vi "Transfer Properties to New Node.vi"(7 "Replacement Channels":T1={"Channel to Replace"="Targets/Controller/Custom Devices/VCOM/CAN_Sender_Tx/ACC/ACC_ESP_E2E_PR2/ACC_NEW_SIGNAL", "Replacement Channel"="Targets/Controller/User Channels/User Channel 1"}, 8 "error in (no error)":errorcluster, 10 "Property Type":i32(ring)=8 items=["K_STRING", "K_BOOL", "K_I32", "K_U32", "K_DOUBLE", "K_U64", "K_VARIANT", "K_DEPENDENTFILE", "K_DEPENDENTNODE", "K_DATASOURCENODE", "K_U16", "K_DBLARR", "K_U32ARR", "K_I32ARR", "K_STRINGARR", "K_DICTIONARY", "K_DICTIONARYARR", "K_BINARYSTRING", "K_I16", "K_I64", "K_BOOLARR", "K_U64ARR", "K_U16ARR", "K_I64ARR", "K_I16ARR"], 11 "reference":refnum<k24>) -> (0 "error out":errorcluster, 2 "Replacement Log":string[](array[string]), 3 "reference out":refnum<k24>)   [LabVIEW 2025]
uses:
  Replacement Channels.ctl
  NationalInstruments.VeriStand.SystemDefinitionAPI
  NationalInstruments.VeriStand.SystemStorage
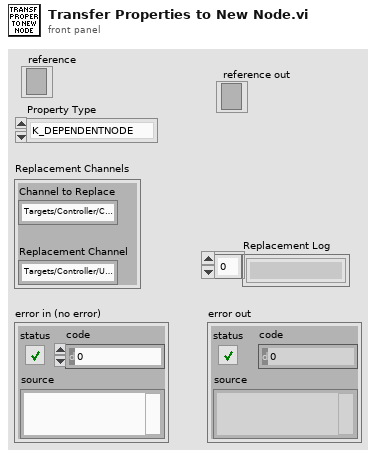
[diagram p1: front panel]
types:
  T1 = typedef "Replacement Channels.ctl" = cluster{"Channel to Replace":string, "Replacement Channel":string}
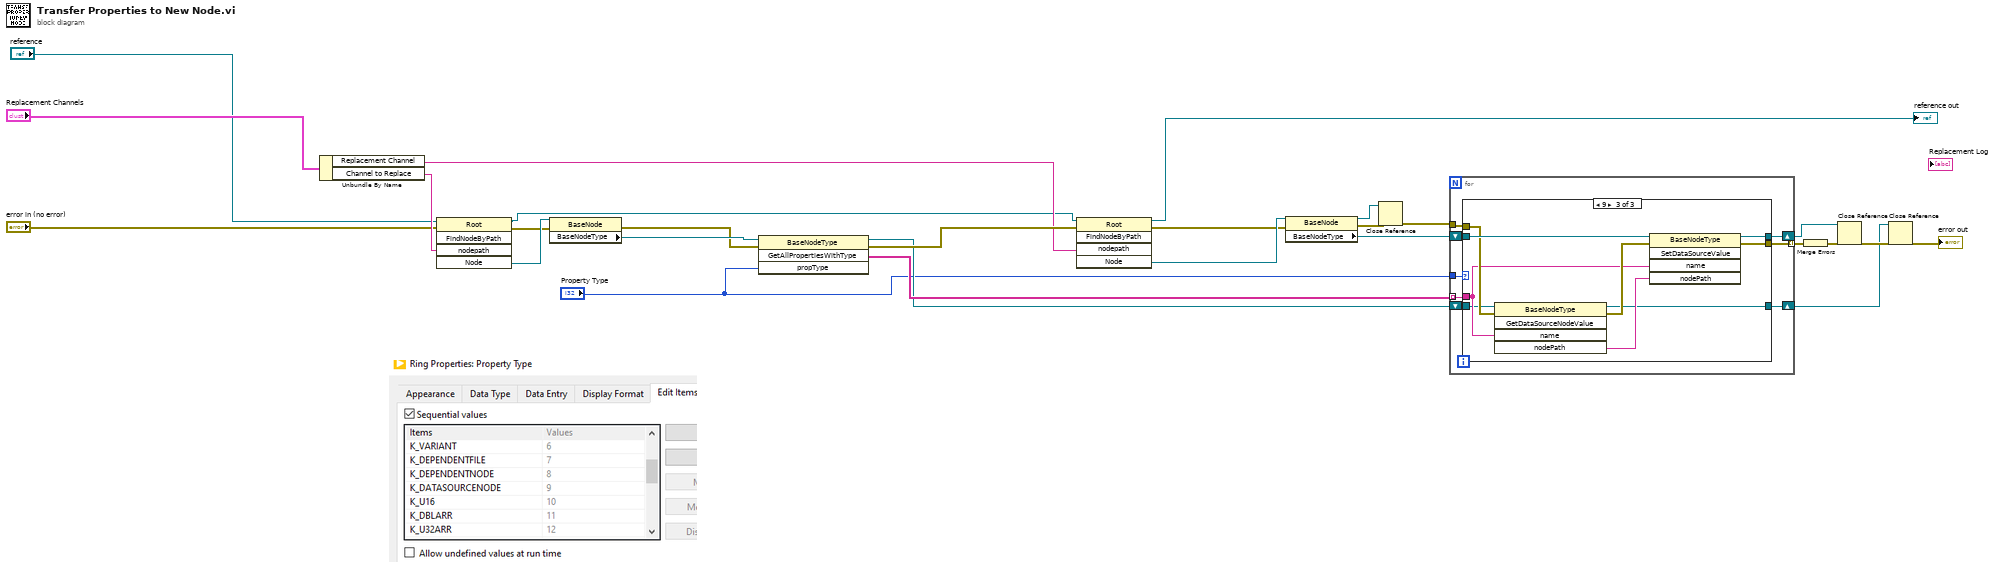
[diagram p0: block diagram]
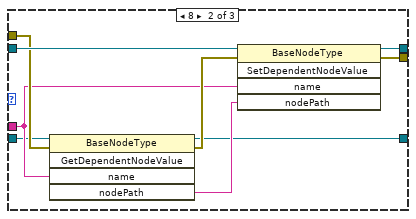
[diagram p3: hidden frame]
diagram:
  n1 = Unbundle By Name("Replacement Channels") -> ("Replacement Channel"=w19:string, "Channel to Replace"=w26:string)
  n2 = invoke class="Root" method="FindNodeByPath"(reference="reference", error in="error in (no error)", "nodepath"=w26) -> (reference out=w3:refnum<k24>, error out=w23:errorcluster, "Node"=w25:refnum<k24>)  [unwired: 2 in, 2 out]
  n3 = property class="BaseNode"(reference=w25, error in=w23) -> (error out=w22:errorcluster, "BaseNodeType"=w24:refnum<k24>)  [unwired: 1 out]
  n4 = invoke class="BaseNodeType" method="GetAllPropertiesWithType"(reference=w24, error in=w22, "propType"="Property Type") -> (reference out=w15:refnum<k24>, error out=w20:errorcluster, "GetAllPropertiesWithType"=w17:string[])  [unwired: 1 in, 1 out]
  n5 = invoke class="Root" method="FindNodeByPath"(reference=w3, error in=w20, "nodepath"=w19) -> (reference out=→"reference out":refnum<k24>, error out=w13:errorcluster, "Node"=w21:refnum<k24>)  [unwired: 2 in, 2 out]
  n6 = property class="BaseNode"(reference=w21, error in=w13) -> (reference out=w11:refnum<k24>, error out=w12:errorcluster, "BaseNodeType"=w18:refnum<k24>)
  n7 = Close Reference(reference=w11, error in (no error)=w12) -> (error out=w10:errorcluster)
  n8 = for {
    tunnel: w10 -> [w34]
    tunnel: w17 -> [w33] mode=indexing
    tunnel: [w32] -> w16 mode=indexing
    tunnel: "Property Type" -> [w30]
    shift-right: [w29] -> w8
    shift-left: w18 -> [w35]
    shift-right: [w28] -> w6
    shift-left: w15 -> [w31]
    n9 = case shown="9" w30 {
      tunnel: w35 -> [w37 w47 w56]
      tunnel: w34 -> [w38 w46 w55]
      tunnel: w33 -> [_ w44 w53]
      tunnel: [w38 w42 w51] -> w32
      tunnel: w31 -> [w36 w41 w50]
      tunnel: [w37 w40 w49] -> w29
      tunnel: [w36 w39 w48] -> w28
      frame 0, Default {
      }
      frame 8 {
        n10 = invoke class="BaseNodeType" method="GetDependentNodeValue"(reference=w41, error in=w46, "name"=w44) -> (reference out=w39:refnum<k24>, error out=w45:errorcluster, "nodePath"=w43:string)  [unwired: 2 in, 2 out]
        n11 = invoke class="BaseNodeType" method="SetDependentNodeValue"(reference=w47, error in=w45, "name"=w44, "nodePath"=w43) -> (reference out=w40:refnum<k24>, error out=w42:errorcluster)  [unwired: 1 in, 3 out]
      }
      frame 9 {
        n12 = invoke class="BaseNodeType" method="GetDataSourceNodeValue"(reference=w50, error in=w55, "name"=w53) -> (reference out=w48:refnum<k24>, error out=w54:errorcluster, "nodePath"=w52:string)  [unwired: 2 in, 2 out]
        n13 = invoke class="BaseNodeType" method="SetDataSourceValue"(reference=w56, error in=w54, "name"=w53, "nodePath"=w52) -> (reference out=w49:refnum<k24>, error out=w51:errorcluster)  [unwired: 1 in, 3 out]
      }
    }
  }
  n14 = Merge Errors(w16) -> (w9:errorcluster)
  n15 = Close Reference(reference=w8, error in (no error)=w9) -> (error out=w7:errorcluster)
  n16 = Close Reference(reference=w6, error in (no error)=w7) -> (error out=→"error out":errorcluster)
